vi "Controll Inputs (SubVI).vi"(7 "Keyboard ID":refnum<k1>, 8 "error in (no error)":errorcluster, 9 "Switch control":bool, 10 "Manual":bool=TRUE, 11 "Controller ID":refnum<k1>) -> (0 "error out":errorcluster, 1 "Land/Take off":bool, 2 "Boolean":bool, 3 "Control cluster":T1)   [LabVIEW 2014]
uses:
  Global.vi
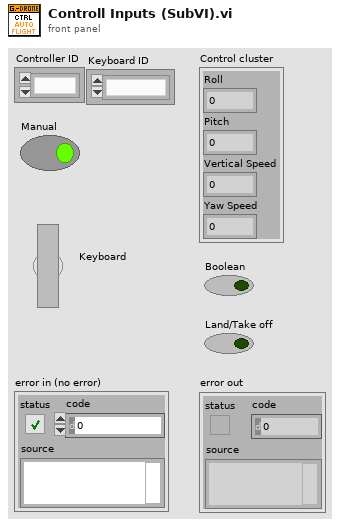
[diagram p1: front panel]
types:
  T1 = cluster{"Roll":dbl, "Pitch":dbl, "Vertical Speed":dbl, "Yaw Speed":dbl}
  T2 = cluster{"Hover":bool, "Land/Take off":bool, "button 3":bool, "button 4":bool}
  T3 = typedef "Control cluster.ctl" = cluster{"Roll":sgl, "Pitch":sgl, "Vertical Speed":sgl, "Yaw Speed":sgl}
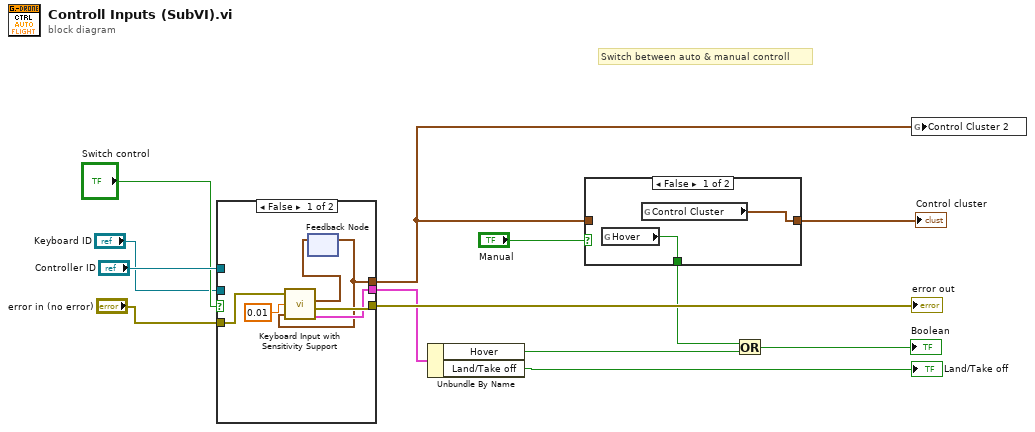
[diagram p0: block diagram]
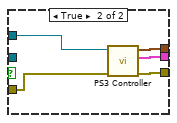
[diagram p2: hidden frame]
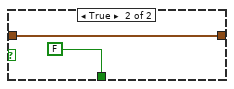
[diagram p3: hidden frame]
diagram:
  # "Switch between auto & manual controll"
  n1 = case shown="False" "Switch control" {
    tunnel: "Controller ID" -> [_ w24]
    tunnel: [w17 w23] -> w12
    tunnel: [w14 w22] -> w11
    tunnel: [w16 w21] -> w1
    tunnel: "error in (no error)" -> [w18 w20]
    tunnel: "Keyboard ID" -> [_ _]
    frame False {
      n2 = feedback #1() -> (w14:T1)  [unwired: 1 in]
      n3 = call "Keyboard Input with Sensitivity Support.vi"("error in (no error)"=w18, "Speed step"=0.01, "Previous Control Cluster"=w14) -> ("Control Cluster"=w15:T1, "error out"=w17:errorcluster, "Buttons control"=w16:T2)  [unwired: 1 in]
      n4 = feedback-in #1(w15) -> ()
    }
    frame True {
      n5 = call "PS3 Controller.vi"("error in (no error)"=w20, "device ID"=w24) -> ("error out"=w23:errorcluster, "Buttons control"=w21:T2, "Control cluster"=w22:T1)  [unwired: 7 in]
    }
  }
  "error out" <- w12
  n6 = Unbundle By Name(w1) -> ("Hover"=w7:bool, "Land/Take off"=→"Land/Take off":bool)
  n7 = case shown="False" "Manual" {
    tunnel: w11 -> [_ w27]
    tunnel: [w26 w27] -> w10
    tunnel: [w25 FALSE] -> w6
    frame False {
      n8 = global read "Global.vi" "Hover"() -> (w25:bool)
      n9 = global read "Global.vi" "Control Cluster"() -> (w26:T3)
    }
    frame True {
    }
  }
  "Control cluster" <- w10
  n10 = Or(x=w6, y=w7) -> (x .or. y?=→"Boolean":bool)
  n11 = global write "Global.vi" "Control Cluster 2"(w11) -> ()
